vi "Get Enumerated List Test Settings.vi"(8 "Error In":errorcluster, 11 "Data Channel Ref In":T1 format="%.0x") -> (0 "Error Out":errorcluster, 2 "Data Channel Settings":T2, 3 "Data Channel Ref Out":T1=18446744073709551615 format="%.0x")   [LabVIEW 2020, in "Instrument Addon Scripting API Channels Unit Tests.lvclass"]
uses:
  Instrument Addon Scripting API Channels Unit Tests.lvclass
  <vilib>/NI VeriStand/Custom Device API/Custom Device Item Ref.ctl
  APIs/Scripting API/TypeDefs/Array Enumerated List Settings.ctl
  APIs/Scripting API/TypeDefs/Array Element.ctl
  <vilib>/NI VeriStand/Custom Device API/Get Item Property (String Array).vi
  <vilib>/NI VeriStand/Custom Device API/Get Item Property (String).vi
  <vilib>/NI VeriStand/Custom Device API/Custom Device API.lvlib
  APIs/Scripting API/Instrument Addon Scripting API.lvlib
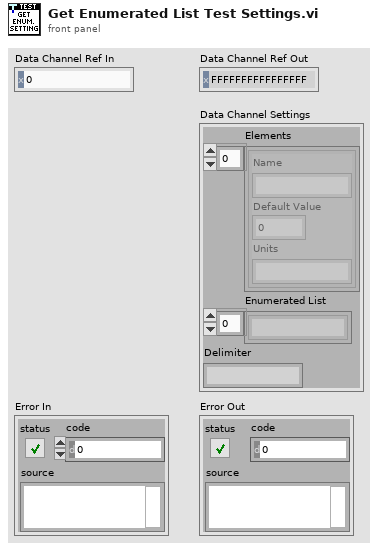
[diagram p1: front panel]
types:
  T1 = typedef "Custom Device API.lvlib/Custom Device Item Ref.ctl" = u64
  T2 = typedef "Instrument Addon Scripting API.lvlib/Array Enumerated List Settings.ctl" = cluster{"Elements":T3[], "Enumerated List":string[], "Delimiter":string}
  T3 = typedef "Instrument Addon Scripting API.lvlib/Array Element.ctl" = cluster{"Name":string, "Default Value":dbl, "Units":string}
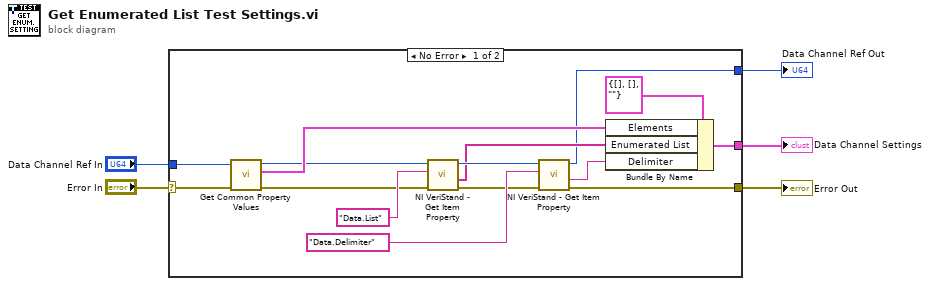
[diagram p0: block diagram]
diagram:
  n1 = case shown="No Error" "Error In" {
    selector: "Error In" -> [w7 w22]
    tunnel: [w20 _] -> w5
    tunnel: [w19 w22] -> w4
    tunnel: "Data Channel Ref In" -> [w9 w21]
    tunnel: [w6 w21] -> w1
    frame No Error {
      n2 = call "Get Common Property Values.vi"("Error In"=w7, "Data Channel  Ref in"=w9) -> ("error out"=w10:errorcluster, "Array Out"=w11:T3[], "Data Channel Ref Out"=w8:u64)  [unwired: 7 in]
      n3 = call-poly <vilib>:"NI VeriStand - Get Item Property.vi"("error in (no error)"=w10, "Property Name"="Data.List", "Item Ref in"=w8) -> ("error out"=w15:errorcluster, "Value"=w14:string[], "Item Ref out"=w16:T1)  [unwired: 5 in, 1 out]
      n4 = call-poly <vilib>:"NI VeriStand - Get Item Property.vi"("error in (no error)"=w15, "Property Name"="Data.Delimiter", "Item Ref in"=w16) -> ("error out"=w19:errorcluster, "Value"=w18:string, "Item Ref out"=w6:T1)  [unwired: 5 in, 1 out]
      n5 = Bundle By Name(cluster=T2 {"Elements"=[], "Enumerated List"=[], "Delimiter"=""} ("Settings"), "Elements"=w11, "Enumerated List"=w14, "Delimiter"=w18) -> (w20:T2)
    }
    frame Error {
    }
  }
  "Data Channel Settings" <- w5
  "Error Out" <- w4
  "Data Channel Ref Out" <- w1
